vi "test-DiffDriveSim-stability.vi"() -> (3 "Test Passed":bool)   [LabVIEW 2019]
uses:
  <vilib>/Rock Robotics/WPI/ThirdParty/JAS_Junk/TrajLib/DCMOTOR.CTL
  <vilib>/Rock Robotics/WPI/ThirdParty/JAS_Junk/TrajLib/LINEAR_SYSTEM.ctl
  <vilib>/Analysis/Matrix/Datatypes/RealMatrix.ctl
  <vilib>/Rock Robotics/WPI/ThirdParty/JAS_Junk/TrajLib/DIFF_DRIVE_TRAIN_SIM.ctl
  <vilib>/Rock Robotics/WPI/ThirdParty/JAS_Junk/TrajLib/DIFF_DRIVE_ToughBoxMini_MotorChoice_ENUM.ctl
  <vilib>/Rock Robotics/WPI/ThirdParty/JAS_Junk/TrajLib/MatBuilder_Create.vi
  <vilib>/Rock Robotics/WPI/ThirdParty/JAS_Junk/TrajLib/LinearSystem_New.vi
  <vilib>/Rock Robotics/WPI/ThirdParty/JAS_Junk/TrajLib/MatBuilder_Fill.vi
  <vilib>/Rock Robotics/WPI/ThirdParty/JAS_Junk/TrajLib/MatrixHelper_Zero.vi
  <vilib>/Rock Robotics/WPI/ThirdParty/JAS_Junk/TrajLib/Util_CalcDist.vi
  <vilib>/Rock Robotics/WPI/ThirdParty/JAS_Junk/TrajLib/MatrixHelper_CoerceSize.vi
  <vilib>/Rock Robotics/WPI/ThirdParty/JAS_Junk/TrajLib/Trajectory_Library.lvlib
  <vilib>/Analysis/Matrix/NI_Matrix.lvlib
panel:
  in  "Tab Control":T1(tab)
  out "Heading Chart":dbl(graph)
  out "Left Motor Vel (PV)":dbl format="%20.3f"
  out "Right Motor Vel (PV)":dbl format="%20.3f"
  out "Motor Amps":cluster{"Voltage":dbl}(graph)
  out "PV Chart":T2(graph)
  out "Motor Amps":dbl format="%20.3f"
  out "Sim Upd Err":bool
  out "Lin Sys Size Cooerced":bool
  out "Pose Norm":dbl
  out "Pos Passed":bool
  out "PV Chart 2":T2(graph)
  out "DiffDriveMotor":T3 {"Jr_KgM2" format="%13.5p"; "L_H" format="%13.5p"; "Kt_NMPerAmp" format="%13.5p"; "KvINV_RadPerSecPerVolt" format="%13.5p"; "R_Ohms" format="%13.5p"; "FreeSpeed_RadPerSec" format="%13.5p"; "FreeCurrent_Amps" format="%13.5p"; "StallCurrent_Amps" format="%13.5p"; "StallTorque_NM" format="%13.5p"; "nominalVoltage_Volts" format="%13.5p"}
  out "m_DiffDriveVel":T4
  out "Differential Drive Train Sim":T6 {"m_Motor"."Jr_KgM2" format="%13.5p"; "m_Motor"."L_H" format="%13.5p"; "m_Motor"."Kt_NMPerAmp" format="%13.5p"; "m_Motor"."KvINV_RadPerSecPerVolt" format="%13.5p"; "m_Motor"."R_Ohms" format="%13.5p"; "m_Motor"."FreeSpeed_RadPerSec" format="%13.5p"; "m_Motor"."FreeCurrent_Amps" format="%13.5p"; "m_Motor"."StallCurrent_Amps" format="%13.5p"; "m_Motor"."StallTorque_NM" format="%13.5p"; "m_Motor"."nominalVoltage_Volts" format="%13.5p"}
  # "<States,States>"
  # "<States,Inputs>"
  # "<Outputs,States>"
  # "<Outputs,Inputs>"
  # "<States, 1>"
  # "<Outputs, 1>"
  # "<Inputs, 1>"
  # "<Outputs, 1>"
  # "<States,States>"
  # "<States,Inputs>"
  # "<Outputs,States>"
  # "<Outputs,Inputs>"
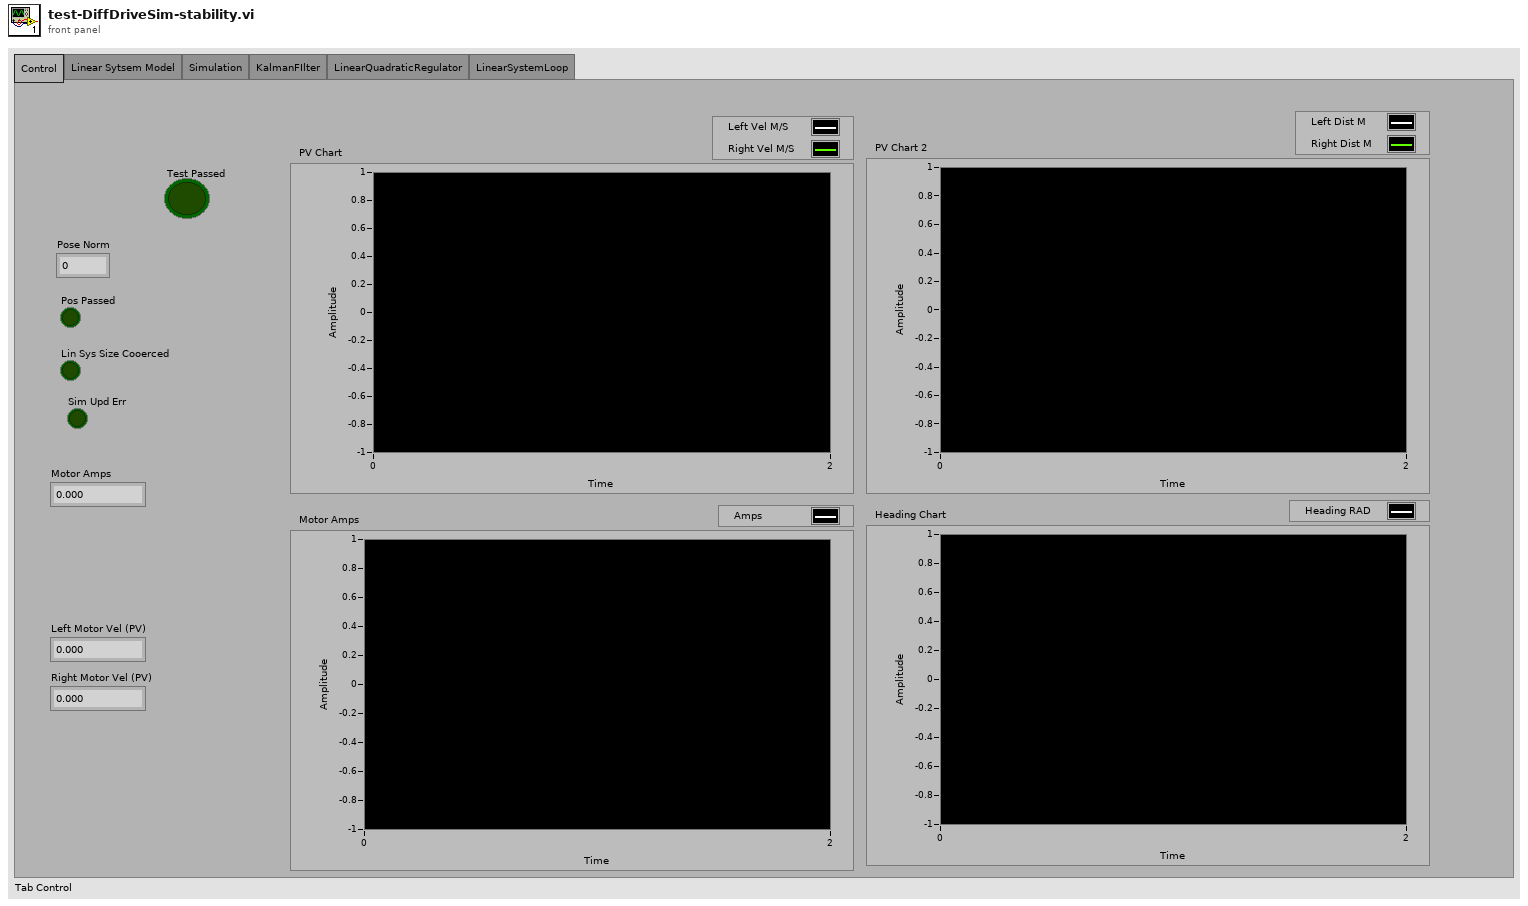
[diagram p1: front panel]
types:
  T1 = enum32{"Control", "Linear Sytsem Model", "Simulation", "KalmanFIlter", "LinearQuadraticRegulator", "LinearSystemLoop"}
  T2 = cluster{"LeftVelocity_M_Per_Sec":dbl, "RightVel_M_Per_Sec":dbl}
  T3 = typedef "Trajectory_Library.lvlib/DCMOTOR.CTL" = cluster{"nominalVoltage_Volts":dbl, "StallTorque_NM":dbl, "StallCurrent_Amps":dbl, "FreeCurrent_Amps":dbl, "FreeSpeed_RadPerSec":dbl, "R_Ohms":dbl, "KvINV_RadPerSecPerVolt":dbl, "Kt_NMPerAmp":dbl, "L_H":dbl, "Jr_KgM2":dbl}
  T4 = typedef "Trajectory_Library.lvlib/LINEAR_SYSTEM.ctl" = cluster{"m_A":T5, "m_B":T5, "m_C":T5, "m_D":T5, "States":i32, "Inputs":i32, "Outputs":i32}
  T5 = typedef "NI_Matrix.lvlib/RealMatrix.ctl" = dbl[][]
  T6 = typedef "Trajectory_Library.lvlib/DIFF_DRIVE_TRAIN_SIM.ctl" = cluster{"m_Plant":T4, "m_X":T5, "m_Y":T5, "m_U":T5, "MeasureStdDev":T5, "m_Motor":T3, "m_OriginalGearing":dbl, "m_CurrentGearing":dbl, "m_WheelRadius_M":dbl, "m_RB":dbl}
  T7 = typedef "Trajectory_Library.lvlib/DIFF_DRIVE_ToughBoxMini_MotorChoice_ENUM.ctl" = enum16{"One CIM Per Side", "Two CIM Per Side", "One MiniCIM Per Side", "Two Mini CIM Per Side", "Two Falcon Per Side", "Two NEO Per Side"}
  T8 = typedef "Trajectory_Library.lvlib/POSE2D.ctl" = cluster{"TRANSLATION":T9, "ROTATION":T10}
  T9 = typedef "Trajectory_Library.lvlib/TRANSLATION2D.ctl" = cluster{"X":dbl, "Y":dbl}
  T10 = typedef "Trajectory_Library.lvlib/ROTATION2D.ctl" = cluster{"VALUE":dbl, "COS":dbl, "SIN":dbl}
  T11 = cluster{"LeftPosition_Meters":dbl, "RightPosition_Meters":dbl}
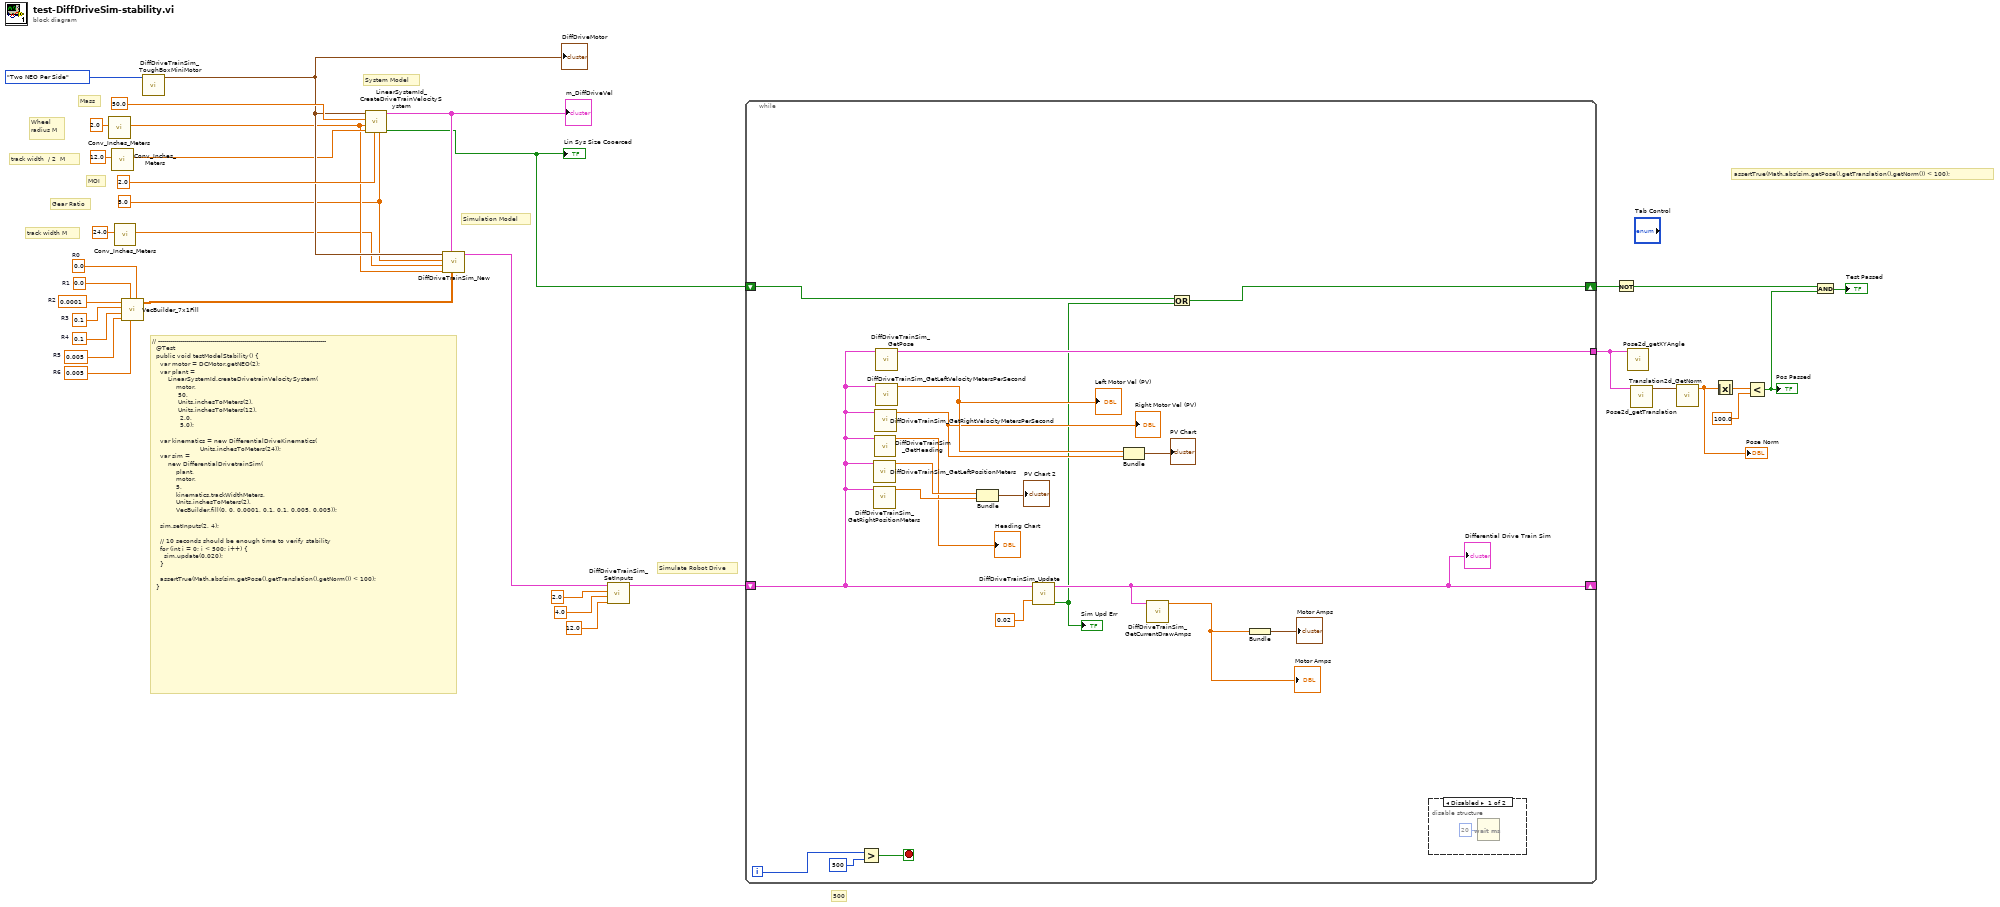
[diagram p0: block diagram]
diagram:
  w23 = 0.005  # R6
  w22 = 0.005  # R5
  w21 = 0.1  # R4
  w20 = 0.1  # R3
  w19 = 0.0001  # R2
  w18 = 0.0  # R1
  w17 = 0.0  # R0
  w26 = 5.0 ("G")
  # "500"
  # "assertTrue(Math.abs(sim.getPose().getTranslation().getNorm()) < 100);"
  # "track width M"
  # "Gear Ratio"
  # "Wheel\nradius M"
  # "track width  / 2  M"
  # "// ------------------------------------------------------------------------------------\n  @Test\n  public void testModelStability() {\n    var motor = DCMotor.getNEO(2);\n    var plant =\n        LinearSystemId.createDrivetrainVelocitySystem(\n            motor, \n             50, \n             Units.inchesToMeters(2), \n             Units.inchesToMeters(12), \n              2.0, \n              5.0);\n\n    var kinematics = new DifferentialDriveKinematics(\n                        Units.inchesToMeters(24));\n    var sim =\n        new DifferentialDrivetrainSim(\n            plant,\n            motor,\n            5,\n            kinematics.trackWidthMeters,\n            Units.inchesToMeters(2),\n            VecBuilder.fill(0, 0, 0.0001, 0.1, 0.1, 0.005, 0.005));\n\n    sim.setInputs(2, 4);\n\n    // 10 seconds should be enough time to verify stability\n    for (int i = 0; i < 500; i++) {\n      sim.update(0.020);\n    }\n\n    assertTrue(Math.abs(sim.getPose().getTranslation().getNorm()) < 100);\n  }"
  # "MOI"
  # "Simulation Model"
  # "System Model"
  # "Mass"
  # "Simulate Robot Drive"
  n1 = call <vilib>:"Conv_Inches_Meters.vi"("INCH"=2.0) -> ("Meters"=w28:dbl)  [unwired: 10 in]
  n2 = call <vilib>:"Conv_Inches_Meters.vi"("INCH"=12.0) -> ("Meters"=w29:dbl)  [unwired: 10 in]
  n3 = call <vilib>:"Conv_Inches_Meters.vi"("INCH"=24.0) -> ("Meters"=w24:dbl)  [unwired: 10 in]
  n4 = call <vilib>:"VecBuilder_7x1Fill.vi"("R0"=w17, "R6"=w23, "R1"=w18, "R5"=w22, "R4"=w21, "R3"=w20, "R2"=w19) -> ("output matrix"=w16:T5)  [unwired: 4 in]
  n5 = call <vilib>:"DiffDriveTrainSim_ToughBoxMiniMotor.vi"("ToughBoxMiniMotor"=DIFF_DRIVE_ToughBoxMini_MotorChoice_ENUM."Two NEO Per Side") -> ("DriveMotor"=w30:T3)  [unwired: 10 in]
  "DiffDriveMotor" <- w30
  n6 = call <vilib>:"LinearSystemId_CreateDriveTrainVelocitySystem.vi"("G"=w26, "JKgMetersSquared"=2.0 ("Mass_Kg"), "rbMeters"=w29, "rMeters"=w28, "MassKg"=50.0 ("Mass_Kg"), "Motor"=w30) -> ("Size Coerced"=w5:bool, "Linearsystem"=w27:T4)  [unwired: 4 in]
  "m_DiffDriveVel" <- w27
  "Lin Sys Size Cooerced" <- w5
  n7 = call <vilib>:"DiffDriveTrainSim_New.vi"("MeasurementStdDev"=w16, "DriveTrainPlant"=w27, "WheelRadius_M"=w28, "TrackWidth_M"=w24, "Gearing"=w26, "DriveMotor"=w30) -> ("DiffDriveTrainSim"=w15:T6)  [unwired: 5 in]
  n8 = call <vilib>:"DiffDriveTrainSim_SetInputs.vi"("BatteryVoltage"=12.0, "Right_Volts"=4.0, "Left_Volts"=2.0, "in DiffDriveTrainSim"=w15) -> ("out DiffDriveTrainSim"=w14:T6)  [unwired: 6 in, 1 out]
  n9 = while {
    shift-right: [w53] -> _
    shift-left: w14 -> [w51]
    tunnel: [w43] -> w10
    shift-right: [w40] -> w4
    shift-left: w5 -> [w41]
    i -> [w49]
    stop <- w47 stop-if-true
    n10 = Greater?(x=w49, y=500) -> (0:w47:bool)
    n11 = call <vilib>:"DiffDriveTrainSim_GetLeftPositionMeters.vi"("DiffDriveTrainSim"=w51) -> ("LeftPosition_Meters"=w38:dbl)  [unwired: 10 in]
    n12 = call <vilib>:"DiffDriveTrainSim_GetRightPositionMeters.vi"("DiffDriveTrainSim"=w51) -> ("RightPosition_Meters"=w37:dbl)  [unwired: 10 in]
    n13 = call <vilib>:"DiffDriveTrainSim_GetHeading.vi"("DiffDriveTrainSim"=w51) -> ("Heading"=→"Heading Chart":dbl)  [unwired: 10 in]
    n14 = call <vilib>:"DiffDriveTrainSim_GetRightVelocityMetersPerSecond.vi"("DiffDriveTrainSim"=w51) -> ("RightVel_M_Per_Sec"=w45:dbl)  [unwired: 10 in]
    "Right Motor Vel (PV)" <- w45
    n15 = call <vilib>:"DiffDriveTrainSim_GetPose.vi"("DiffDriveTrainSim"=w51) -> ("Pose"=w43:T8)  [unwired: 10 in]
    n16 = call <vilib>:"DiffDriveTrainSim_GetLeftVelocityMetersPerSecond.vi"("DiffDriveTrainSim"=w51) -> ("LeftVelocity_M_Per_Sec"=w52:dbl)  [unwired: 10 in]
    "Left Motor Vel (PV)" <- w52
    n17 = Bundle("LeftPosition_Meters"=w38, "RightPosition_Meters"=w37) -> (→"PV Chart 2":T11)  [unwired: 1 in]
    n18 = call <vilib>:"DiffDriveTrainSim_Update.vi"("dT_Seconds"=0.02, "in DiffDriveTrainSim"=w51) -> ("Error"=w42:bool, "out DiffDriveTrainSim"=w53:T6)  [unwired: 8 in]
    "Sim Upd Err" <- w42
    "Differential Drive Train Sim" <- w53
    n19 = Bundle("LeftVelocity_M_Per_Sec"=w52, "RightVel_M_Per_Sec"=w45) -> (→"PV Chart":T2)  [unwired: 1 in]
    n20 = call <vilib>:"DiffDriveTrainSim_GetCurrentDrawAmps.vi"("DiffDriveTrainSim"=w53) -> ("TotalCurrent_Amps"=w46:dbl)  [unwired: 10 in]
    "Motor Amps" <- w46
    n21 = Or(x=w41, y=w42) -> (x .or. y?=w40:bool)
    n22 = Bundle("TotalCurrent_Amps"=w46) -> (→"Motor Amps":cluster{"TotalCurrent_Amps":dbl})  [unwired: 1 in]
    n23 = disable-structure shown="Disabled" {
      frame Disabled {
        n24 = Wait (ms)(milliseconds to wait=u32 20) -> ()  [unwired: 1 out]
      }
      frame Enabled {
      }
    }
  }
  n25 = Not(x=w4) -> (.not. x?=w3:bool)
  n26 = call <vilib>:"Pose2d_getXYAngle.vi"("in POSE"=w10) -> ()  [unwired: 8 in, 3 out]
  n27 = call <vilib>:"Pose2d_getTranslation.vi"("in POSE"=w10) -> ("outTRANSLATION"=w9:T9)  [unwired: 10 in]
  n28 = call <vilib>:"Translation2d_GetNorm.vi"("In Translation"=w9) -> ("Norm"=w8:dbl)  [unwired: 10 in]
  "Pose Norm" <- w8
  n29 = Absolute Value(x=w8) -> (abs(x)=w7:dbl)
  n30 = Less?(x=w7, y=100.0) -> (x < y?=w2:bool)
  "Pos Passed" <- w2
  n31 = And(x=w3, y=w2) -> (x .and. y?=→"Test Passed":bool)
